vi "Out_S2F15.vi"(8 "error in (no error)":errorcluster, 10 "S2F15":T1, 11 "S2 Message Class in":refnum<class "S2 Message Class.lvclass">) -> (0 "error out":errorcluster, 3 "S2 Message Class out":refnum<class "S2 Message Class.lvclass">)   [LabVIEW 2020, in "SECS Communication.lvlib" / "S2 Message Class.lvclass"]
uses:
  S2 Message Class.lvclass
  D:/Dropbox/SECS/SECS_GEM v1.0.6/Com/SECS Communication/SECS-II Class/SECS-II Class.lvclass
  S2F15.ctl
  SECS-II Class/Format Code.ctl
  SECS-II Class/Data Message_List.vi
  SECS-II Class/Data Message_U4.vi
  SECS-II Class/Variant To Data_ASCII.vi
  SECS-II Class/Data Message_ASCII.vi
  SECS-II Class/Variant To Data_Binary.vi
  SECS-II Class/Data Message_Binary.vi
  SECS-II Class/Variant To Data_Boolean.vi
  SECS-II Class/Data Message_Boolean.vi
  SECS-II Class/Variant To Data_J.vi
  SECS-II Class/Data Message_J.vi
  SECS-II Class/Variant To Data_I1.vi
  SECS-II Class/Data Message_I1 .vi
  SECS-II Class/Variant To Data_I2.vi
  SECS-II Class/Data Message_I2.vi
  SECS-II Class/Variant To Data_I4.vi
  SECS-II Class/Data Message_I4.vi
  SECS-II Class/Variant To Data_I8.vi
  SECS-II Class/Data Message_I8.vi
  SECS-II Class/Variant To Data_U1.vi
  SECS-II Class/Data Message_U1.vi
  SECS-II Class/Variant To Data_U2.vi
  SECS-II Class/Data Message_U2.vi
  SECS-II Class/Variant To Data_U4.vi
  SECS-II Class/Variant To Data_U8.vi
  SECS-II Class/Data Message_U8.vi
  SECS-II Class/Variant To Data_F4.vi
  SECS-II Class/Data Message_F4.vi
  SECS-II Class/Variant To Data_F8.vi
  SECS-II Class/Data Message_F8.vi
  SECS-II Class/Variant To Data_Character.vi
  SECS-II Class/Data Message_Character.vi
  SECS-II Class/SECS-II Class.lvclass
  D:/Dropbox/SECS/SECS_GEM v1.0.6/Com/SECS Communication/S2 Message Class/S2 Message Class.lvclass
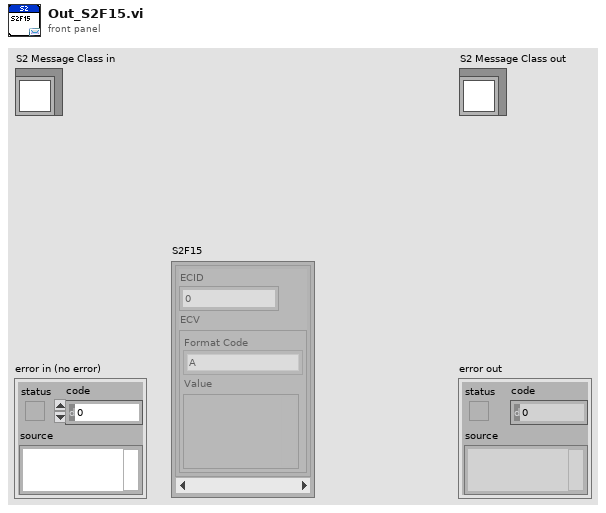
[diagram p1: front panel]
types:
  T1 = typedef "SECS Communication.lvlib/S2 Message Class.lvclass/S2F15.ctl" = cluster{"ECID":u32, "ECV":cluster{"Format Code":T2, "Value":variant}}[]
  T2 = typedef "SECS Communication.lvlib/SECS-II Class.lvclass/Format Code.ctl" = enum16{"L", "A", "B", "Boolean", "J", "I1", "I2", "I4", "I8", "U1", "U2", "U4", "U8", "F4", "F8", "Char"}
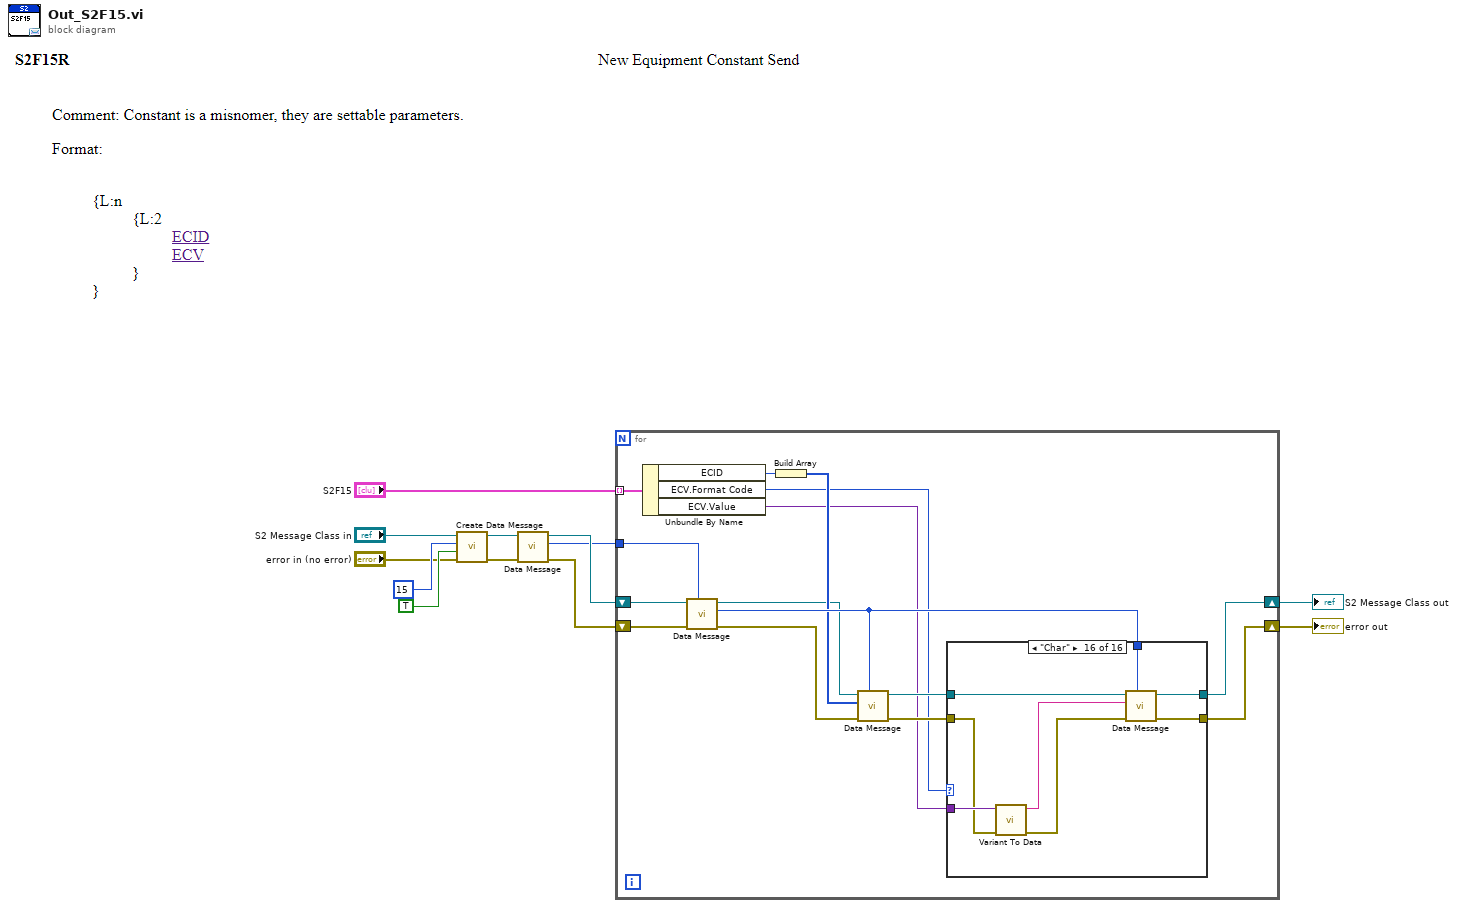
[diagram p0: block diagram]
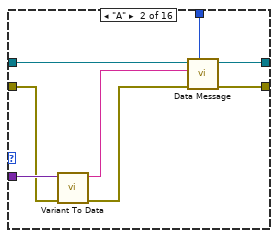
[diagram p3: hidden frame]
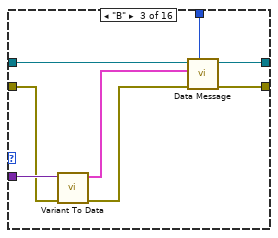
[diagram p4: hidden frame]
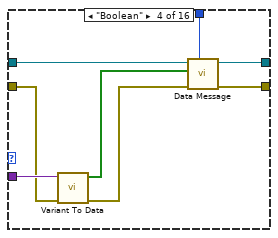
[diagram p5: hidden frame]
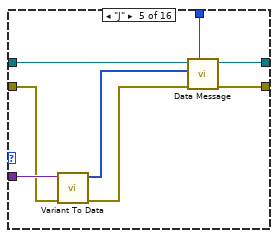
[diagram p6: hidden frame]
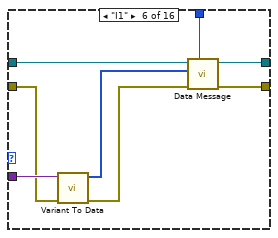
[diagram p7: hidden frame]
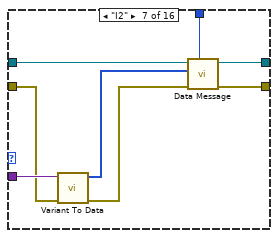
[diagram p8: hidden frame]
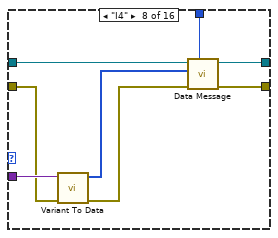
[diagram p9: hidden frame]
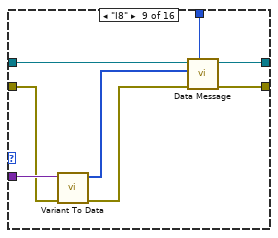
[diagram p10: hidden frame]
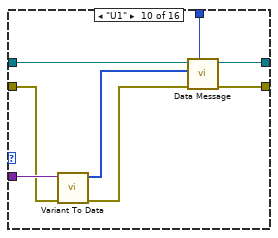
[diagram p11: hidden frame]
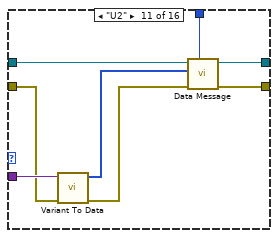
[diagram p12: hidden frame]
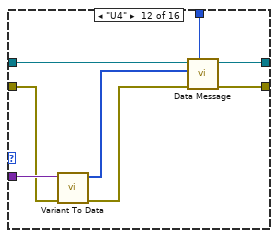
[diagram p13: hidden frame]
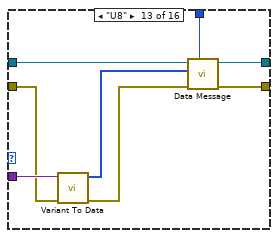
[diagram p14: hidden frame]
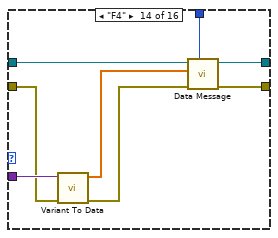
[diagram p15: hidden frame]
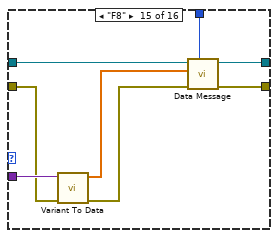
[diagram p16: hidden frame]
diagram:
  n1 = call "Create Data Message.vi"("error in (no error)"="error in (no error)", "W-Bit"=TRUE, "Function"=u8 15, "SECS-II Class in"="S2 Message Class in") -> ("error out"=w9:errorcluster, "SECS-II Class out"=w10:refnum<class "S2 Message Class.lvclass">)  [unwired: 6 in]
  n2 = call-poly "Data Message.vi"("error in"=w9, "SECS-II Class in"=w10) -> ("error out"=w5:errorcluster, "Index"=w3:i32, "SECS-II Class out"=w6:refnum<class "S2 Message Class.lvclass">)  [unwired: 7 in]
  n3 = for {
    shift-right: [w14] -> w1
    shift-left: w6 -> [w26]
    shift-right: [w13] -> w2
    shift-left: w5 -> [w27]
    tunnel: "S2F15" -> [w24] mode=indexing
    tunnel: w3 -> [w25]
    n4 = Unbundle By Name(w24) -> ("ECID"=w19:u32, "ECV.Format Code"=w16:T2, "ECV.Value"=w15:variant)
    n5 = call-poly "Data Message.vi"("Parent Index"=w25, "error in"=w27, "SECS-II Class in"=w26) -> ("error out"=w21:errorcluster, "Index"=w20:i32, "SECS-II Class out"=w17:refnum<class "S2 Message Class.lvclass">)  [unwired: 6 in]
    n6 = Build Array(w19) -> (w18:u32[])
    n7 = call-poly "Data Message.vi"("Parent Index"=w20, "error in"=w21, "Data"=w18, "SECS-II Class in"=w17) -> ("error out"=w22:errorcluster, "SECS-II Class out"=w23:refnum<class "S2 Message Class.lvclass">)  [unwired: 6 in]
    n8 = case shown="\"Char\"" w16 {
      tunnel: w15 -> [_ w33 w41 w49 w57 w65 w73 w81 w89 w97 w105 w113 w121 w129 w137 w145]
      tunnel: w23 -> [w29 w37 w45 w53 w61 w69 w77 w85 w93 w101 w109 w117 w125 w133 w141 w149]
      tunnel: w22 -> [w28 w32 w40 w48 w56 w64 w72 w80 w88 w96 w104 w112 w120 w128 w136 w144]
      tunnel: [w29 w35 w43 w51 w59 w67 w75 w83 w91 w99 w107 w115 w123 w131 w139 w147] -> w14
      tunnel: [w28 w34 w42 w50 w58 w66 w74 w82 w90 w98 w106 w114 w122 w130 w138 w146] -> w13
      tunnel: w20 -> [_ w36 w44 w52 w60 w68 w76 w84 w92 w100 w108 w116 w124 w132 w140 w148]
      frame "L", Default {
      }
      frame "A" {
        n9 = call-poly "Variant To Data.vi"("error in (no error)"=w32, "Variant"=w33) -> ("error out"=w31:errorcluster, "Data"=w30:string)  [unwired: 7 in, 1 out]
        n10 = call-poly "Data Message.vi"("Parent Index"=w36, "error in"=w31, "Data"=w30, "SECS-II Class in"=w37) -> ("error out"=w34:errorcluster, "SECS-II Class out"=w35:refnum<class "S2 Message Class.lvclass">)  [unwired: 6 in]
      }
      frame "B" {
        n11 = call-poly "Variant To Data.vi"("error in (no error)"=w40, "Variant"=w41) -> ("error out"=w39:errorcluster, "Data Cluster"=w38:cluster{"Data":bool[]}[])  [unwired: 7 in, 1 out]
        n12 = call-poly "Data Message.vi"("Parent Index"=w44, "error in"=w39, "Data Cluster"=w38, "SECS-II Class in"=w45) -> ("error out"=w42:errorcluster, "SECS-II Class out"=w43:refnum<class "S2 Message Class.lvclass">)  [unwired: 6 in]
      }
      frame "Boolean" {
        n13 = call-poly "Variant To Data.vi"("error in (no error)"=w48, "Variant"=w49) -> ("error out"=w47:errorcluster, "Data"=w46:bool[])  [unwired: 7 in, 1 out]
        n14 = call-poly "Data Message.vi"("Parent Index"=w52, "error in"=w47, "Data"=w46, "SECS-II Class in"=w53) -> ("error out"=w50:errorcluster, "SECS-II Class out"=w51:refnum<class "S2 Message Class.lvclass">)  [unwired: 6 in]
      }
      frame "J" {
        n15 = call-poly "Variant To Data.vi"("error in (no error)"=w56, "Variant"=w57) -> ("error out"=w55:errorcluster, "Data"=w54:i64[])  [unwired: 7 in, 1 out]
        n16 = call-poly "Data Message.vi"("Parent Index"=w60, "error in"=w55, "Data"=w54, "SECS-II Class in"=w61) -> ("error out"=w58:errorcluster, "SECS-II Class out"=w59:refnum<class "S2 Message Class.lvclass">)  [unwired: 6 in]
      }
      frame "I1" {
        n17 = call-poly "Variant To Data.vi"("error in (no error)"=w64, "Variant"=w65) -> ("error out"=w63:errorcluster, "Data"=w62:i8[])  [unwired: 7 in, 1 out]
        n18 = call-poly "Data Message.vi"("Parent Index"=w68, "error in"=w63, "Data"=w62, "SECS-II Class in"=w69) -> ("error out"=w66:errorcluster, "SECS-II Class out"=w67:refnum<class "S2 Message Class.lvclass">)  [unwired: 6 in]
      }
      frame "I2" {
        n19 = call-poly "Variant To Data.vi"("error in (no error)"=w72, "Variant"=w73) -> ("error out"=w71:errorcluster, "Data"=w70:i16[])  [unwired: 7 in, 1 out]
        n20 = call-poly "Data Message.vi"("Parent Index"=w76, "error in"=w71, "Data"=w70, "SECS-II Class in"=w77) -> ("error out"=w74:errorcluster, "SECS-II Class out"=w75:refnum<class "S2 Message Class.lvclass">)  [unwired: 6 in]
      }
      frame "I4" {
        n21 = call-poly "Variant To Data.vi"("error in (no error)"=w80, "Variant"=w81) -> ("error out"=w79:errorcluster, "Data"=w78:i32[])  [unwired: 7 in, 1 out]
        n22 = call-poly "Data Message.vi"("Parent Index"=w84, "error in"=w79, "Data"=w78, "SECS-II Class in"=w85) -> ("error out"=w82:errorcluster, "SECS-II Class out"=w83:refnum<class "S2 Message Class.lvclass">)  [unwired: 6 in]
      }
      frame "I8" {
        n23 = call-poly "Variant To Data.vi"("error in (no error)"=w88, "Variant"=w89) -> ("error out"=w87:errorcluster, "Data"=w86:i64[])  [unwired: 7 in, 1 out]
        n24 = call-poly "Data Message.vi"("Parent Index"=w92, "error in"=w87, "Data"=w86, "SECS-II Class in"=w93) -> ("error out"=w90:errorcluster, "SECS-II Class out"=w91:refnum<class "S2 Message Class.lvclass">)  [unwired: 6 in]
      }
      frame "U1" {
        n25 = call-poly "Variant To Data.vi"("error in (no error)"=w96, "Variant"=w97) -> ("error out"=w95:errorcluster, "Data"=w94:u8[])  [unwired: 7 in, 1 out]
        n26 = call-poly "Data Message.vi"("Parent Index"=w100, "error in"=w95, "Data"=w94, "SECS-II Class in"=w101) -> ("error out"=w98:errorcluster, "SECS-II Class out"=w99:refnum<class "S2 Message Class.lvclass">)  [unwired: 6 in]
      }
      frame "U2" {
        n27 = call-poly "Variant To Data.vi"("error in (no error)"=w104, "Variant"=w105) -> ("error out"=w103:errorcluster, "Data"=w102:u16[])  [unwired: 7 in, 1 out]
        n28 = call-poly "Data Message.vi"("Parent Index"=w108, "error in"=w103, "Data"=w102, "SECS-II Class in"=w109) -> ("error out"=w106:errorcluster, "SECS-II Class out"=w107:refnum<class "S2 Message Class.lvclass">)  [unwired: 6 in]
      }
      frame "U4" {
        n29 = call-poly "Variant To Data.vi"("error in (no error)"=w112, "Variant"=w113) -> ("error out"=w111:errorcluster, "Data"=w110:u32[])  [unwired: 7 in, 1 out]
        n30 = call-poly "Data Message.vi"("Parent Index"=w116, "error in"=w111, "Data"=w110, "SECS-II Class in"=w117) -> ("error out"=w114:errorcluster, "SECS-II Class out"=w115:refnum<class "S2 Message Class.lvclass">)  [unwired: 6 in]
      }
      frame "U8" {
        n31 = call-poly "Variant To Data.vi"("error in (no error)"=w120, "Variant"=w121) -> ("error out"=w119:errorcluster, "Data"=w118:u64[])  [unwired: 7 in, 1 out]
        n32 = call-poly "Data Message.vi"("Parent Index"=w124, "error in"=w119, "Data"=w118, "SECS-II Class in"=w125) -> ("error out"=w122:errorcluster, "SECS-II Class out"=w123:refnum<class "S2 Message Class.lvclass">)  [unwired: 6 in]
      }
      frame "F4" {
        n33 = call-poly "Variant To Data.vi"("error in (no error)"=w128, "Variant"=w129) -> ("error out"=w127:errorcluster, "Data"=w126:sgl[])  [unwired: 7 in, 1 out]
        n34 = call-poly "Data Message.vi"("Parent Index"=w132, "error in"=w127, "Data"=w126, "SECS-II Class in"=w133) -> ("error out"=w130:errorcluster, "SECS-II Class out"=w131:refnum<class "S2 Message Class.lvclass">)  [unwired: 6 in]
      }
      frame "F8" {
        n35 = call-poly "Variant To Data.vi"("error in (no error)"=w136, "Variant"=w137) -> ("error out"=w135:errorcluster, "Data"=w134:dbl[])  [unwired: 7 in, 1 out]
        n36 = call-poly "Data Message.vi"("Parent Index"=w140, "error in"=w135, "Data"=w134, "SECS-II Class in"=w141) -> ("error out"=w138:errorcluster, "SECS-II Class out"=w139:refnum<class "S2 Message Class.lvclass">)  [unwired: 6 in]
      }
      frame "Char" {
        n37 = call-poly "Variant To Data.vi"("error in (no error)"=w144, "Variant"=w145) -> ("error out"=w143:errorcluster, "Data"=w142:string)  [unwired: 7 in, 1 out]
        n38 = call-poly "Data Message.vi"("Parent Index"=w148, "error in"=w143, "Data"=w142, "SECS-II Class in"=w149) -> ("error out"=w146:errorcluster, "SECS-II Class out"=w147:refnum<class "S2 Message Class.lvclass">)  [unwired: 6 in]
      }
    }
  }
  "error out" <- w2
  "S2 Message Class out" <- w1
